vi "Pixel 4 Condition (SubVI).vi"(8 "Image Width":u16=240, 10 "Contour Scan in":T1, 11 "Fnd?":bool) -> (2 "Contour Scan out":T1)   [LabVIEW 2015]
uses:
  Controls (FPGA)/Contour Scan.ctl
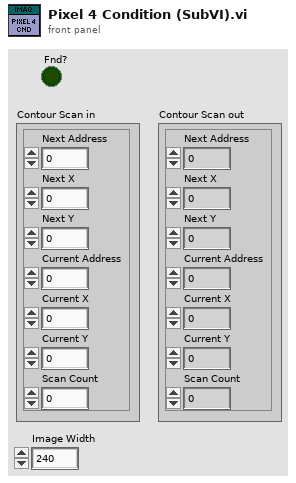
[diagram p1: front panel]
types:
  T1 = typedef "Contour Scan.ctl" = cluster{"Next Address":fxp<+,24,24>, "Next X":fxp<+,12,12>, "Next Y":fxp<+,12,12>, "Current Address":fxp<+,24,24>, "Current X":fxp<+,12,12>, "Current Y":fxp<+,12,12>, "Scan Count":u32}
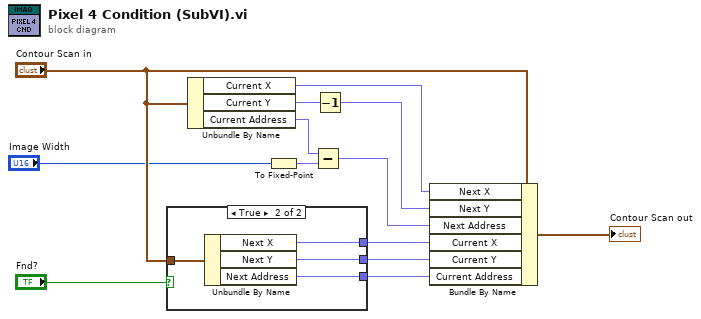
[diagram p0: block diagram]
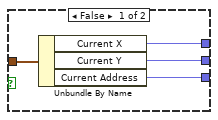
[diagram p2: hidden frame]
diagram:
  n1 = case shown="True" "Fnd?" {
    tunnel: "Contour Scan in" -> [w17 w21]
    tunnel: [w16 w20] -> w11
    tunnel: [w15 w19] -> w12
    tunnel: [w14 w18] -> w13
    frame False {
      n2 = Unbundle By Name(w17) -> ("Current X"=w16:fxp<+,12,12>, "Current Y"=w15:fxp<+,12,12>, "Current Address"=w14:fxp<+,24,24>)
    }
    frame True {
      n3 = Unbundle By Name(w21) -> ("Next X"=w20:fxp<+,12,12>, "Next Y"=w19:fxp<+,12,12>, "Next Address"=w18:fxp<+,24,24>)
    }
  }
  n4 = Unbundle By Name("Contour Scan in") -> ("Current X"=w8:fxp<+,12,12>, "Current Y"=w6:fxp<+,12,12>, "Current Address"=w2:fxp<+,24,24>)
  n5 = To Fixed-Point(number="Image Width") -> (fixed-point=w4:fxp<+,12,12>)  [unwired: 1 in]
  n6 = Subtract(x=w2, y=w4) -> (x-y=w3:fxp<+,24,24>)
  n7 = Decrement(x=w6) -> (x-1=w5:fxp<+,12,12>)
  n8 = Bundle By Name(cluster="Contour Scan in", "Next X"=w8, "Next Y"=w5, "Next Address"=w3, "Current X"=w11, "Current Y"=w12, "Current Address"=w13) -> (→"Contour Scan out":T1)
